vi "subGeneratePackets.vi"(0 "Message Text":string, 4 "Message Type":bool, 5 "PSK system parameters":T2, 6 "Packet Parameters":T1, 7 "Packet Pad \n[samples]":i32, 8 "PN sequence order\nfor Sync Bits":i32, 9 "Pulse Shaping Filter Parameters":T3, 10 "Tx IQ Sampling\nRate [s/sec]":dbl, 11 "Samples per Symbol":i32) -> (1 "Symbol Rate":dbl, 2 "Packets":cluster{"t0":dbl, "dt":dbl, "Y":cdb[]}[](array[cluster]), 3 "Number of Packets":i32)   [LabVIEW 2013]
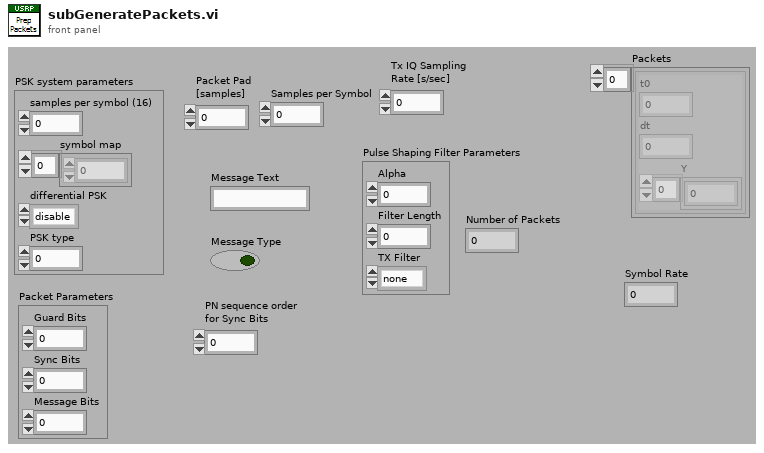
[diagram p1: front panel]
types:
  T1 = cluster{"Guard Bits ":i32, "Sync Bits":i32, "Message Bits":i32}
  T2 = cluster{"samples per symbol (16)":i32, "symbol map":cdb[], "differential PSK":enum16{"disable", "enable"}, "PSK type":u16}
  T3 = cluster{"Alpha":dbl, "Filter Length":i32, "TX Filter":enum16{"none", "Raised Cosine", "Root Raised Cos", "Gaussian"}}
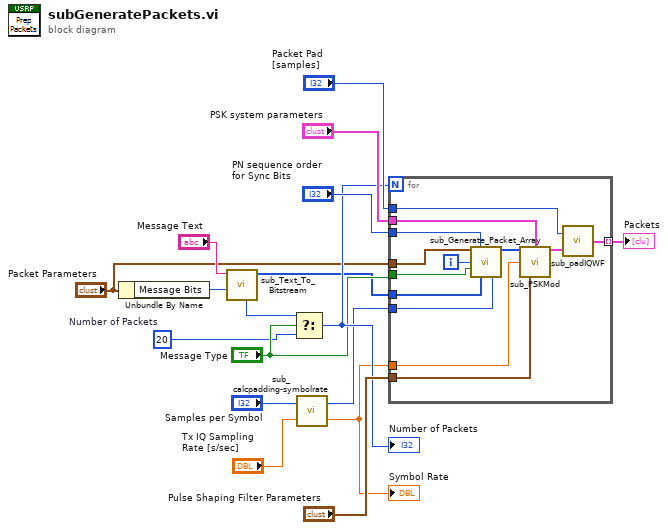
[diagram p0: block diagram]
diagram:
  w10 = 20  # Number of Packets
  n1 = Unbundle By Name("Packet Parameters") -> ("Message Bits"=w5:i32)
  n2 = call "sub_Text_To_Bitstream.vi"("Packet\nMessage Length (bits)"=w5, "text"="Message Text") -> ("message bitstream"=w9:i8[], "Number of Packets"=w12:i32)  [unwired: 7 in, 1 out]
  n3 = Select(t=w12, s="Message Type", f=w10) -> (s? t:f=w13:i32)
  "Number of Packets" <- w13
  n4 = call "sub_calcpadding-symbolrate.vi"("Tx IQ Sampling\nRate [s/sec]"="Tx IQ Sampling\nRate [s/sec]", "Samples per Symbol"="Samples per Symbol") -> ("Symbol Rate"=w2:dbl, "Padding Bits"=w4:i32)
  "Symbol Rate" <- w2
  n5 = for {
    N: w13 -> [_]
    tunnel: "Packet Parameters" -> [w27]
    tunnel: [w20] -> w7 mode=indexing
    tunnel: "Message Type" -> [w29]
    tunnel: w9 -> [w28]
    tunnel: "PN sequence order\nfor Sync Bits" -> [w26]
    tunnel: w4 -> [w25]
    tunnel: "PSK system parameters" -> [w23]
    tunnel: w2 -> [w22]
    tunnel: "Pulse Shaping Filter Parameters" -> [w21]
    tunnel: "Packet Pad \n[samples]" -> [w18]
    i -> [w30]
    n6 = call "sub_Generate_Packet_Array.vi"("Packet Parameters"=w27, "PN sequence order\nfor Sync"=w26, "Packet Number"=w30, "User defined bitstream?"=w29, "user  bitstream"=w28, "Cyclic Padding Bits"=w25) -> ("Output Packet"=w24:i8[])  [unwired: 9 in]
    n7 = call "sub_PSKMod.vi"("Packet to Transmit"=w24, "PSK system parameters"=w23, "Symbol Rate, Hz"=w22, "filter parameters"=w21) -> ("output complex waveform"=w19:cluster{"t0":dbl, "dt":dbl, "Y":cdb[]})  [unwired: 9 in, 2 out]
    n8 = call "sub_padIQWF.vi"("input complex waveform"=w19, "Packet Pad \n[samples]"=w18) -> ("output complex waveform"=w20:cluster{"t0":dbl, "dt":dbl, "Y":cdb[]})
  }
  "Packets" <- w7
